vi "C_format_file.vi"(8 "error in (no error)":errorcluster, 10 "Format File":enum16{"TXT", "TDMS"}(ring), 11 "Contador_Bin_Actor in":refnum<class "Contador_Bin_Actor.lvclass">) -> (0 "error out":errorcluster, 3 "Contador_Bin_Actor out":refnum<class "Contador_Bin_Actor.lvclass">)   [LabVIEW 2019, in "Contador_Bin_Actor.lvlib" / "Contador_Bin_Actor.lvclass"]
uses:
  Contador_Bin_Actor.lvclass
  C:/Program Files/National Instruments/LabVIEW 2019/vi.lib/ActorFramework/Actor/Actor.lvclass
  Contador_Bin_Actor.lvclass/Contador_Bin_Actor.ctl
  Logging_Contador_Actor/Logging_Contador_Actor/Logging_Contador_Actor.lvclass
  Logging_Contador_Actor_TDMS/Logging_Contador_Actor_TDMS/Logging_Contador_Actor_TDMS.lvclass
  C:/Users/Luis/Documents/Ingenieria/Git_versiones/Actor-framework-CML-con-opciones-de-adquisici-n-main/Logging_Contador_Actor/Logging_Contador_Actor/Logging_Contador_Actor.lvclass
  <vilib>/ActorFramework/Message Enqueuer/Message Enqueuer.lvclass/Message Enqueuer.ctl
  <vilib>/ActorFramework/Message Enqueuer/Enqueue.vi
  <vilib>/ActorFramework/Stop Msg/Stop Msg.lvclass
  C:/Program Files/National Instruments/LabVIEW 2019/vi.lib/ActorFramework/Message/Message.lvclass
  <vilib>/ActorFramework/Message Priority Queue/Priority Enqueue.vi
  <vilib>/ActorFramework/Actor/Actor.lvclass
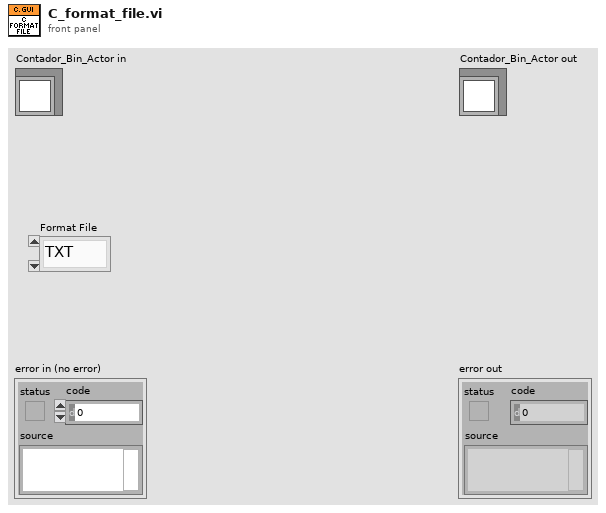
[diagram p1: front panel]
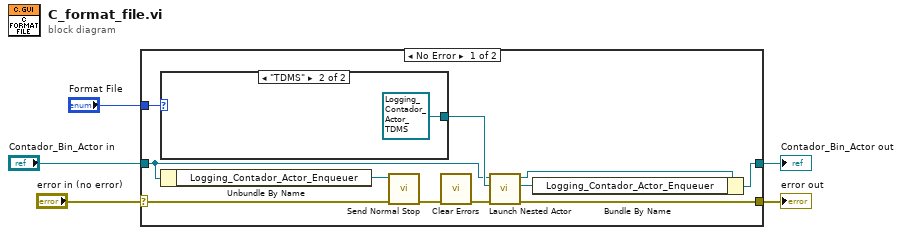
[diagram p0: block diagram]
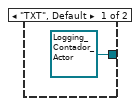
[diagram p2: hidden frame]
diagram:
  n1 = case shown="No Error" "error in (no error)" {
    selector: "error in (no error)" -> [w8 w20]
    tunnel: [w9 w20] -> w4
    tunnel: [w14 w19] -> w2
    tunnel: "Contador_Bin_Actor in" -> [w7 w19]
    tunnel: "Format File" -> [w16 _]
    frame No Error {
      n2 = case shown="\"TDMS\"" w16 {
        tunnel: [refnum<class "Logging_Contador_Actor.lvclass"> refnum ("Logging_Contador_Actor.lvlib:Logging_Contador_Actor.lvclass") refnum<class "Logging_Contador_Actor_TDMS.lvclass"> refnum ("Logging_Contador_Actor_TDMS.lvlib:Logging_Contador_Actor_TDMS.lvclass")] -> w15
        frame "TXT", Default {
        }
        frame "TDMS" {
        }
      }
      n3 = Unbundle By Name(w7) -> ("Logging_Contador_Actor_Enqueuer"=w10:refnum<class "Message Enqueuer.lvclass">)
      n4 = call <vilib>:"Send Normal Stop.vi"("error in (no error)"=w8, "Message Enqueuer"=w10) -> ("error out"=w12:errorcluster)  [unwired: 9 in]
      n5 = call <vilib>:"Clear Errors.vi"("error in (no error)"=w12) -> ("error out"=w6:errorcluster)  [unwired: 5 in, 1 out]
      n6 = call <vilib>:"Launch Nested Actor.vi"("error in (no error)"=w6, "Nested Actor"=w15, "Caller Actor in"=w7) -> ("error out"=w9:errorcluster, "Nested Actor's Enqueuer"=w13:refnum<class "Message Enqueuer.lvclass">, "Caller Actor out"=w11:refnum<class "Contador_Bin_Actor.lvclass">)  [unwired: 6 in]
      n7 = Bundle By Name(cluster=w11, "Logging_Contador_Actor_Enqueuer"=w13) -> (w14:refnum<class "Contador_Bin_Actor.lvclass">)
    }
    frame Error {
    }
  }
  "error out" <- w4
  "Contador_Bin_Actor out" <- w2
